vi "MH_T2 Read Acq QueueBack.vi"() -> ()   [LabVIEW 2019]
uses:
  <userlib>/MultiHarp150/T2Lib/MH_T2QMessage.ctl
  <userlib>/MultiHarp150/T2Lib/MH_T2DeltaQMessage.ctl
panel:
  out "sortie d'erreur":errorcluster caption="ErrorOut"
  out "RollOver":bool
  in  "BufSze":i32=1000000
  in  "entrée d'erreur":errorcluster caption="ErrorIn"
  in  "WIndowW":u32
  in  "Save Data":bool
  in  "Correl Ch":u32=2
  in  "Base Ch":u32=1
  in  "refnum":refnum<file>
  out "DeltaT":u32[](array[numeric])
  out "nActual":i32[](array[numeric])
  out "En Attente":i32[](array[numeric])
  out "Tableau":u64[][](array[numeric])
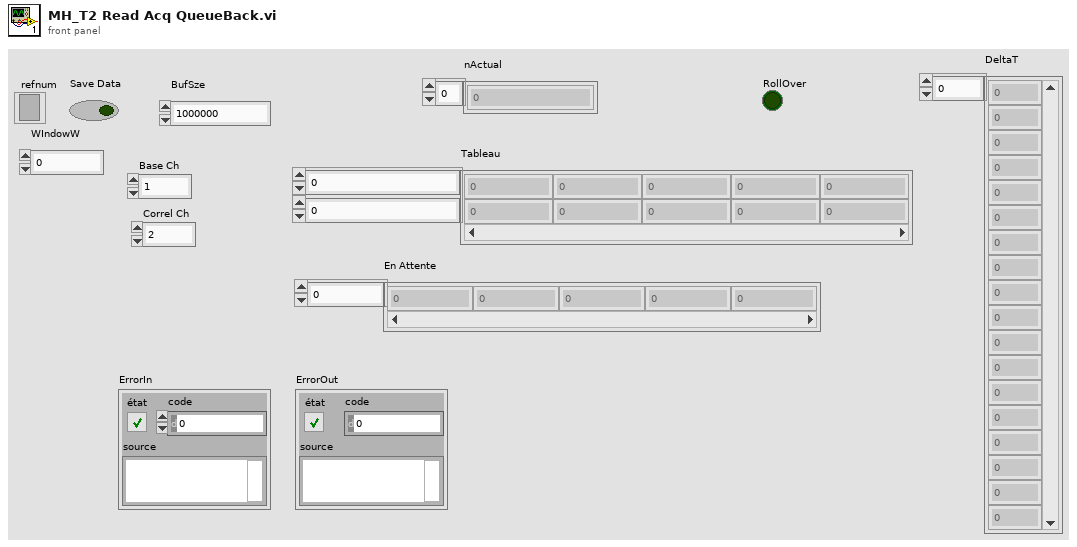
[diagram p1: front panel]
types:
  T1 = typedef "MH_T2DeltaQMessage.ctl" = cluster{"Message":string, "buffer":i32[], "Code":i32, "nactual":i32}
  T2 = typedef "MH_T2QMessage.ctl" = cluster{"Message":string, "buffer":u32[], "Code":i32, "nactual":i32}
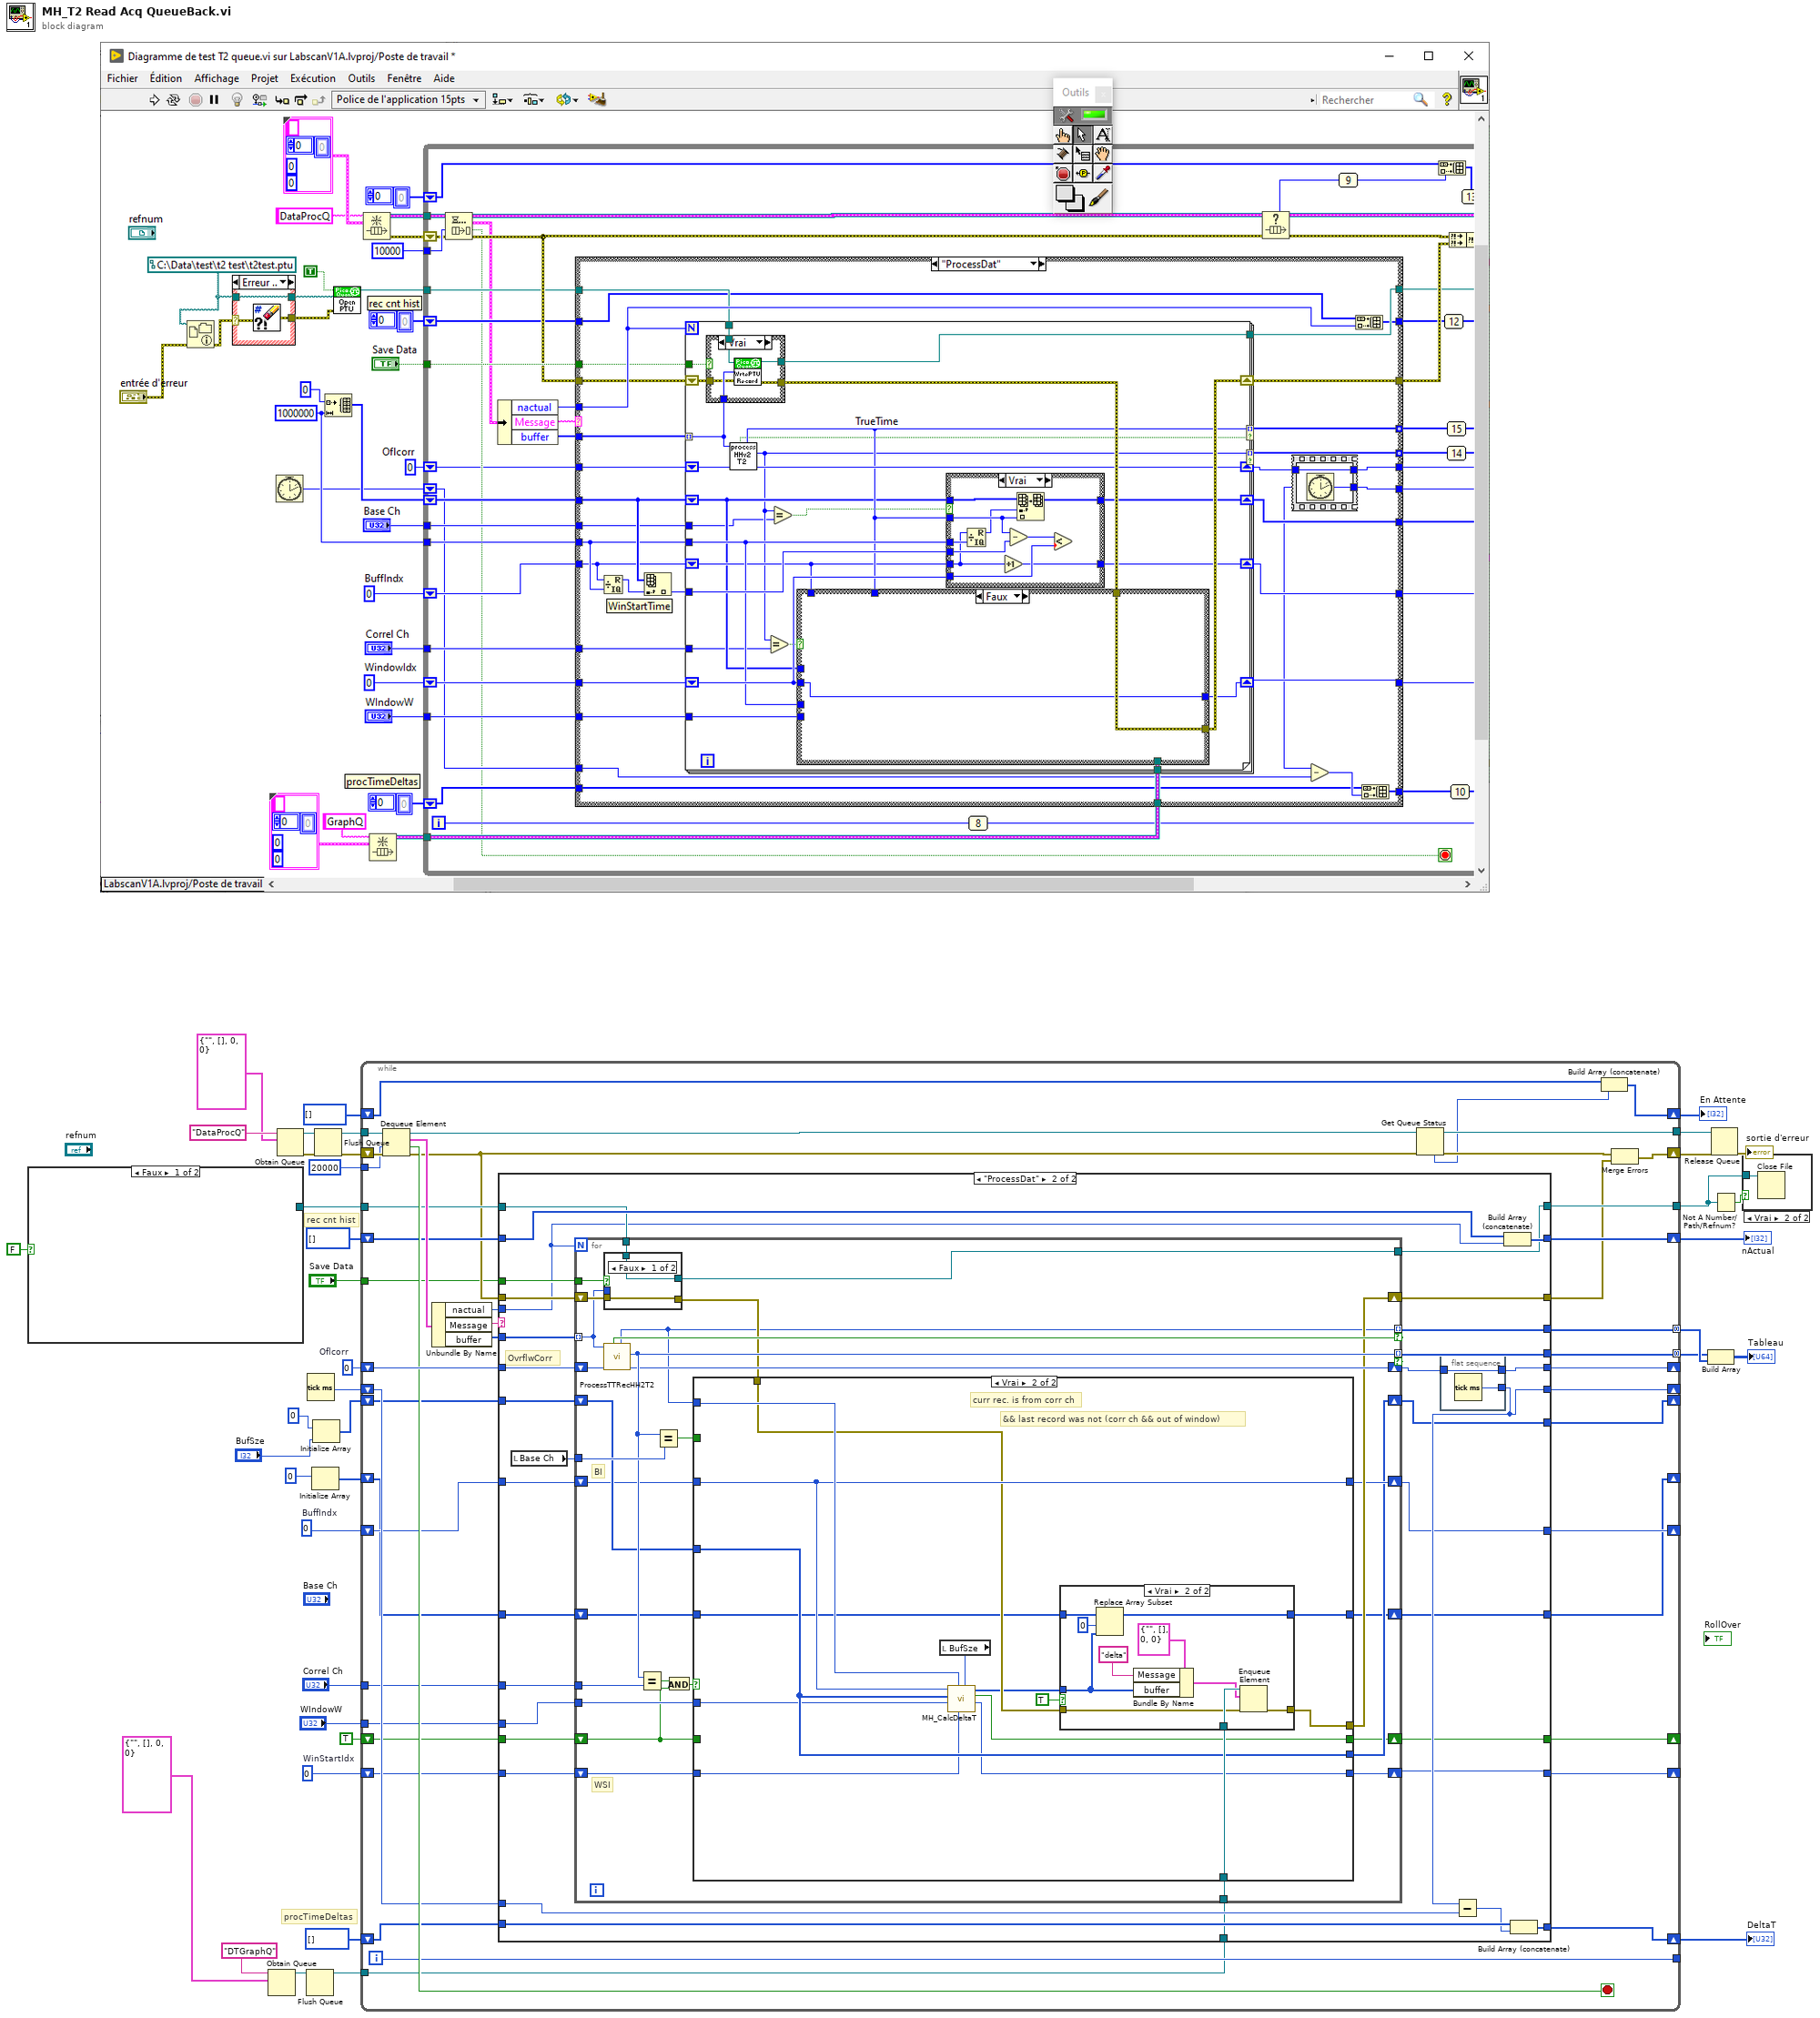
[diagram p0: block diagram]
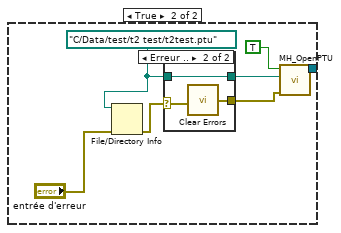
[diagram p3: hidden frame]
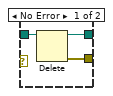
[diagram p4: hidden frame]
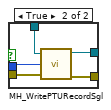
[diagram p6: hidden frame]
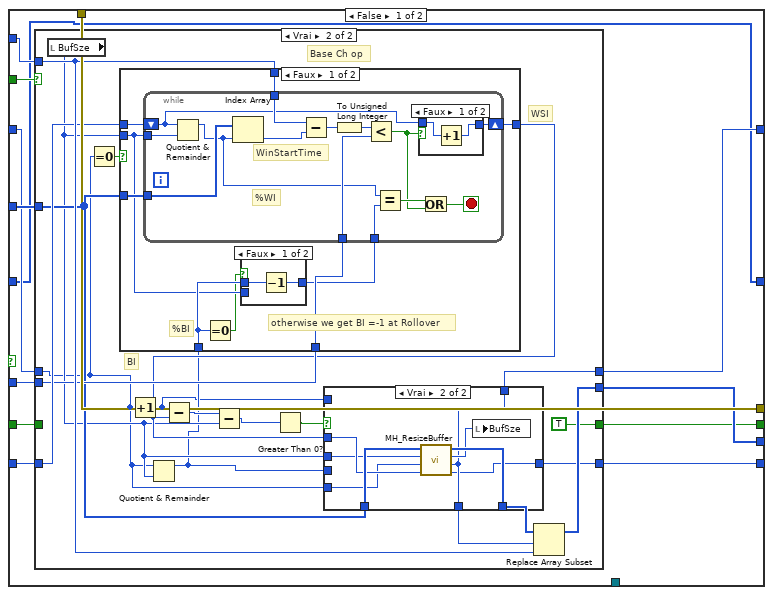
[diagram p7: hidden frame]
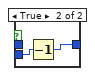
[diagram p9: hidden frame]
diagram:
  w20 = 0  # WinStartIdx
  w8 = 0  # BuffIndx
  w38 = u64 0  # Oflcorr
  # "procTimeDeltas"
  # "rec cnt hist"
  n1 = case shown="Faux" FALSE {
    tunnel: [_ w46] -> w25
    frame False {
    }
    frame True {
      w43 = path "C:/Data/test/t2 test/t2test.ptu" ("chemin sélectionné")
      n2 = File/Directory Info(path=w43, error in="entrée d'erreur") -> (error out=w42:errorcluster)  [unwired: 6 out]
      n3 = case shown="Erreur .." w42 {
        selector: w42 -> [_ w52]
        tunnel: w43 -> [w50 w53]
        tunnel: [w49 w53] -> w45
        tunnel: [w48 w51] -> w44
        frame No Error {
          n4 = Delete(path (use dialog)=w50) -> (deleted path=w49:path, error out=w48:errorcluster)  [unwired: 4 in, 1 out]
        }
        frame Error {
          n5 = call <vilib>:"Clear Errors.vi"("error in (no error)"=w52) -> ("error out"=w51:errorcluster)  [unwired: 5 in, 1 out]
        }
      }
      n6 = call <userlib>:"MH_OpenPTU.vi"("ErrorIn"=w44, "chemin sélectionné"=w45, "WriteMode"=TRUE) -> ("refnum en sortie"=w46:refnum<file>)  [unwired: 6 in, 2 out]
    }
  }
  n7 = Obtain Queue(name (unnamed)="DTGraphQ" ("nom (aucun)"), element data type=T1 {"Message"="", "buffer"=[], "Code"=0, "nactual"=0} ("ClassQueue")) -> (queue out=w16:refnum<queue>)  [unwired: 3 in, 2 out]
  n8 = Obtain Queue(name (unnamed)="DataProcQ" ("nom (aucun)"), element data type=T2 {"Message"="", "buffer"=[], "Code"=0, "nactual"=0} ("ClassQueue")) -> (queue out=w5:refnum<queue>, error out=w2:errorcluster)  [unwired: 3 in, 1 out]
  n9 = Flush Queue(queue=w16) -> (queue out=w10:refnum<queue>)  [unwired: 1 in, 2 out]
  n10 = Tick Count (ms)() -> (millisecond timer value=w31:u32)
  n11 = Initialize Array(u32 0 ("truetime")) -> (w6:u32[])  [unwired: 1 in]
  n12 = Initialize Array(u64 0 ("truetime"), "BufSze") -> (w22:u64[])
  n13 = Flush Queue(queue=w5, error in (no error)=w2) -> (queue out=w4:refnum<queue>, error out=w3:errorcluster)  [unwired: 1 out]
  n14 = while {
    tunnel: w4 -> [w96]
    shift-right: [w72] -> w37
    shift-left: w3 -> [w97]
    shift-right: [w94] -> _
    shift-left: w38 -> [w95]
    tunnel: [w93] -> w34 mode=concatenating
    tunnel: [w89] -> _
    tunnel: [w85] -> w36
    tunnel: [w84] -> w33 mode=concatenating
    shift-right: [w82] -> _
    shift-left: w31 -> [w83]
    shift-right: [w80] -> w29
    shift-left: u32[] [] ("DeltaT") -> [w81]
    shift-right: [w78] -> w27
    shift-left: i32[] [] ("DeltaT") -> [w79]
    shift-right: [w76] -> w35
    shift-left: i32[] [] ("DeltaT") -> [w75]
    tunnel: w25 -> [w74]
    tunnel: [w71] -> w13
    tunnel: "Save Data" -> [w70]
    shift-right: [w65] -> _
    shift-left: w22 -> [w69]
    shift-right: [w67] -> _
    shift-left: w8 -> [w68]
    tunnel: "Correl Ch" -> [w66]
    shift-right: [w61] -> _
    shift-left: w20 -> [w64]
    tunnel: "WIndowW" -> [w63]
    tunnel: 20000 ("timeout en ms (-1)") -> [w62]
    tunnel: w10 -> [w59]
    shift-right: [w57] -> _
    shift-left: TRUE -> [w56]
    shift-right: [w54] -> _
    shift-left: w6 -> [w55]
    i -> [w89]
    stop <- w91 stop-if-true
    n15 = Dequeue Element(queue=w96, timeout in ms (-1)=w62, error in (no error)=w97) -> (queue out=w87:refnum<queue>, element=w92:T2, timed out?=w91:bool, error out=w73:errorcluster)
    n16 = Unbundle By Name(w92) -> ("nactual"=w60:i32, "Message"=w88:string, "buffer"=w90:u32[])
    n17 = case shown="\"ProcessDat\"" w88 {
      tunnel: w95 -> [w108 w141]
      tunnel: [w108 w138] -> w94
      tunnel: [_ w140] -> w93
      tunnel: w90 -> [_ w130]
      tunnel: [_ w139] -> w84
      tunnel: w83 -> [w107 w131]
      tunnel: [w106 w135] -> w80
      tunnel: [w107 w132] -> w82
      tunnel: w81 -> [w106 w137]
      tunnel: w79 -> [w105 w134]
      tunnel: [w105 w133] -> w78
      tunnel: w74 -> [w104 w129]
      tunnel: w73 -> [w100 w128]
      tunnel: [w104 w127] -> w71
      tunnel: w70 -> [_ w126]
      tunnel: w69 -> [w102 w114]
      tunnel: w68 -> [w103 w115]
      tunnel: [w103 w124] -> w67
      tunnel: w66 -> [_ w125]
      tunnel: [w102 w123] -> w65
      tunnel: w64 -> [w101 w122]
      tunnel: w63 -> [_ w121]
      tunnel: [w101 w119] -> w61
      tunnel: w60 -> [_ w118]
      tunnel: w59 -> [_ w117]
      tunnel: [w100 w116] -> w58
      tunnel: [w99 w112] -> w57
      tunnel: w56 -> [w99 w111]
      tunnel: w55 -> [w98 w110]
      tunnel: [w98 w109] -> w54
      frame "Faux", Default {
      }
      frame "ProcessDat" {
        # "OvrflwCorr"
        n18 = local read "Base Ch"() -> (w113:u32)
        n19 = for {
          N: w118 -> [_]
          tunnel: [w152] -> w140 mode=indexing if=w171
          tunnel: w130 -> [w166] mode=indexing
          tunnel: [w164] -> w139 mode=indexing if=w171
          tunnel: w113 -> [w170]
          tunnel: w129 -> [w169]
          tunnel: [w167] -> w127
          tunnel: w126 -> [w165]
          shift-right: [w149] -> w123
          shift-left: w114 -> [w153]
          shift-right: [w150] -> w124
          shift-left: w115 -> [w151]
          tunnel: w125 -> [w162]
          tunnel: w121 -> [w161]
          shift-right: [w160] -> w120
          shift-left: w141 -> [w172]
          shift-right: [w159] -> w119
          shift-left: w122 -> [w155]
          shift-right: [w156] -> w116
          shift-left: w128 -> [w168]
          tunnel: w117 -> [w158]
          shift-right: [w148] -> w112
          shift-left: w111 -> [w146]
          shift-right: [w144] -> w109
          shift-left: w110 -> [w145]
          # "BI"
          # "WSI"
          n20 = case shown="Faux" w165 {
            tunnel: w169 -> [w173 w179]
            tunnel: w168 -> [w174 w178]
            tunnel: [w173 w177] -> w167
            tunnel: [w174 w176] -> w157
            tunnel: w166 -> [_ w175]
            frame False {
            }
            frame True {
              n21 = call <userlib>:"MH_WritePTURecordSgl.vi"("refnum"=w179, "TTTR Records"=w175, "error in"=w178) -> ("refnum en sortie"=w177:refnum<file>, "error out"=w176:errorcluster)  [unwired: 6 in]
            }
          }
          n22 = call <userlib>:"ProcessTTRecHH2T2.vi"("oflcorr_in"=w172, "rawbits"=w166) -> ("oflcorr_out"=w160:u64, "channel"=w164:u32, "truetime"=w152:u64, "is_photon"=w171:bool)  [unwired: 4 in, 2 out]
          n23 = Equal?(x=w164, y=w162) -> (x = y?=w163:bool)
          n24 = Equal?(x=w164, y=w170) -> (x = y?=w154:bool)
          n25 = And(x=w163, y=w146) -> (x .and. y?=w147:bool)
          n26 = case shown="Vrai" w147 {
            tunnel: w153 -> [w190 w271]
            tunnel: w155 -> [w186 w266]
            tunnel: w151 -> [w188 w268]
            tunnel: w161 -> [w184 w267]
            tunnel: [w183 w264] -> w159
            tunnel: w158 -> [_ w273]
            tunnel: w157 -> [w192 w263]
            tunnel: [w192 w272] -> w156
            tunnel: w154 -> [w189 _]
            tunnel: w152 -> [w185 w270]
            tunnel: [w187 w268] -> w150
            tunnel: [w191 w271] -> w149
            tunnel: [w182 w265] -> w148
            tunnel: w146 -> [w181 _]
            tunnel: w145 -> [w180 w260]
            tunnel: [w180 w259] -> w144
            frame False {
              n27 = case shown="Vrai" w189 {
                tunnel: w190 -> [w195 w209]
                tunnel: w185 -> [_ w214]
                tunnel: w188 -> [w196 w200]
                tunnel: [w196 w204] -> w187
                tunnel: [w195 w215] -> w191
                tunnel: w186 -> [w194 w213]
                tunnel: w184 -> [_ w212]
                tunnel: [w194 w203] -> w183
                tunnel: [w193 TRUE] -> w182
                tunnel: w181 -> [w193 _]
                frame False {
                  # "could be sync or non-relevant channel or last ch was (corr ch && out of window)"
                }
                frame True {
                  # "WSI"
                  # "Base Ch op"
                  # "BI"
                  n28 = local read "BufSze"() -> (w202:i32)
                  n29 = Equal To 0?(x=w200) -> (x = 0?=w199:bool)
                  n30 = Increment(x=w200) -> (x+1=w198:i32)
                  n31 = Quotient & Remainder(x=w200, y=w202) -> (x-y*floor(x/y)=w201:i32)  [unwired: 1 out]
                  n32 = case shown="Faux" w199 {
                    tunnel: w214 -> [w224 _]
                    tunnel: w213 -> [w223 w246]
                    tunnel: w212 -> [w222 _]
                    tunnel: w209 -> [w221 _]
                    tunnel: [w220 w246] -> w206
                    tunnel: w202 -> [w217 _]
                    tunnel: w201 -> [w219 _]
                    frame False {
                      # "otherwise we get BI =-1 at Rollover"
                      # "%BI"
                      n33 = Equal To 0?(x=w219) -> (x = 0?=w216:bool)
                      n34 = case shown="Faux" w216 {
                        tunnel: w219 -> [w226 _]
                        tunnel: [w225 w227] -> w218
                        tunnel: w217 -> [_ w228]
                        frame False {
                          n35 = Decrement(x=w226) -> (x-1=w225:i32)
                        }
                        frame True {
                          n36 = Decrement(x=w228) -> (x-1=w227:i32)
                        }
                      }
                      n37 = while {
                        tunnel: w217 -> [w233]
                        tunnel: w224 -> [w242]
                        tunnel: w221 -> [w241]
                        shift-right: [w229] -> w220
                        shift-left: w223 -> [w230]
                        tunnel: w222 -> [w238]
                        tunnel: w218 -> [w232]
                        stop <- w236 stop-if-true
                        # "%WI"
                        # "WinStartTime"
                        n38 = Quotient & Remainder(x=w230, y=w233) -> (x-y*floor(x/y)=w234:i32)  [unwired: 1 out]
                        n39 = Index Array(array=w241, index=w234) -> (element=w240:u64)
                        n40 = Subtract(x=w242, y=w240) -> (x-y=w239:u64)
                        n41 = To Unsigned Long Integer(number=w239) -> (unsigned 32bit integer=w237:u32)
                        n42 = Less?(x=w237, y=w238) -> (x < y?=w231:bool)
                        n43 = Equal?(x=w234, y=w232) -> (x = y?=w235:bool)
                        n44 = case shown="Faux" w231 {
                          tunnel: w230 -> [w244 w245]
                          tunnel: [w243 w245] -> w229
                          frame False {
                            n45 = Increment(x=w244) -> (x+1=w243:i32)
                          }
                          frame True {
                          }
                        }
                        n46 = Or(x=w235, y=w231) -> (x .or. y?=w236:bool)
                      }
                    }
                    frame True {
                    }
                  }
                  n47 = Subtract(x=w198, y=w206) -> (x-y=w211:i32)
                  n48 = Subtract(x=w211, y=w202) -> (x-y=w210:i32)
                  n49 = Greater Than 0?(x=w210) -> (x > 0?=w207:bool)
                  n50 = case shown="Vrai" w207 {
                    tunnel: w209 -> [w250 w258]
                    tunnel: w202 -> [_ w256]
                    tunnel: [w250 w254] -> w208
                    tunnel: w200 -> [_ w255]
                    tunnel: w206 -> [w249 w257]
                    tunnel: [w248 w252] -> w205
                    tunnel: [w247 w252] -> w204
                    tunnel: [w249 w251] -> w203
                    tunnel: w201 -> [w248 _]
                    tunnel: w198 -> [w247 _]
                    frame False {
                    }
                    frame True {
                      n51 = call <userlib>:"MH_ResizeBuffer.vi"("Buffindex"=w257, "Buffsize"=w255, "WinIndex"=w256, "Tableau"=w258) -> ("NewBuffsize"=w251:i32, "NewBuffIndex"=w252:i32, "NewWinIndex"=w253:i32, "tableau (n rotations)"=w254:u64[])  [unwired: 2 in, 2 out]
                      n52 = local write "BufSze"(w253) -> ()
                    }
                  }
                  n53 = Replace Array Subset(array=w208, new element=w214, index=w205) -> (w215:u64[])
                }
              }
            }
            frame True {
              # "&& last record was not (corr ch && out of window)"
              # "curr rec. is from corr ch"
              n54 = local read "BufSze"() -> (w269:i32)
              n55 = call <userlib>:"MH_CalcDeltaT.vi"("Buffsize"=w269, "WinIndex"=w266, "TrueTime"=w270, "WIndowW"=w267, "Data In"=w271, "Buffindex"=w268) -> ("WinIndexOut"=w264:i32, "NewDelta"=w265:bool, "DeltaT Out"=w262:i32[])  [unwired: 3 in]
              n56 = case shown="Vrai" TRUE {
                tunnel: w262 -> [_ w278]
                tunnel: w273 -> [_ w284]
                tunnel: [w275 w283] -> w272
                tunnel: w263 -> [w275 w282]
                tunnel: w260 -> [w274 w281]
                tunnel: [w274 w280] -> w259
                frame False {
                  # "The 2 last records delta T>window"
                  # "we didnt add any deltaT"
                }
                frame True {
                  n57 = Replace Array Subset(array=w281, new element=w278, index=0 ("indice")) -> (w280:u32[])
                  n58 = Bundle By Name(cluster=T1 {"Message"="", "buffer"=[], "Code"=0, "nactual"=0} ("élément"), "Message"="delta", "buffer"=w278) -> (w276:T1)
                  n59 = Enqueue Element(queue=w284, element=w276, error in (no error)=w282) -> (error out=w283:errorcluster)  [unwired: 1 in, 2 out]
                }
              }
            }
          }
        }
        n60 = flat-sequence {
          tunnel: [w143] -> w138
          tunnel: w120 -> [w143]
          tunnel: [w142] -> w132
          frame #0 {
            n61 = Tick Count (ms)() -> (millisecond timer value=w142:u32)
          }
        }
        n62 = Subtract(x=w132, y=w131) -> (x-y=w136:u32)
        n63 = Build Array (concatenate)(w134, w118) -> (w133:i32[])
        n64 = Build Array (concatenate)(w137, w136) -> (w135:u32[])
      }
    }
    n65 = Get Queue Status(queue=w87, error in (no error)=w73) -> (queue out=w85:refnum<queue>, error out=w86:errorcluster, # elements in queue=w77:i32)  [unwired: 1 in, 5 out]
    n66 = Build Array (concatenate)(w75, w77) -> (w76:i32[])
    n67 = Merge Errors(w86, w58) -> (w72:errorcluster)
  }
  "En Attente" <- w35
  "nActual" <- w27
  "DeltaT" <- w29
  n68 = Build Array(w33, w34) -> (→"Tableau":u64[][])
  n69 = Release Queue(queue=w36, error in (no error)=w37) -> (error out=→"sortie d'erreur":errorcluster)  [unwired: 1 in, 2 out]
  n70 = Not A Number/Path/Refnum?(number/path/refnum=w13) -> (NaN/Path/Refnum?=w12:bool)
  n71 = case shown="Vrai" w12 {
    tunnel: w13 -> [_ w286]
    frame False {
    }
    frame True {
      n72 = Close File(refnum=w286) -> ()  [unwired: 1 in, 2 out]
    }
  }
